vi "Get Child Channels.vi"(7 "Channel Type":T1, 8 "error in":errorcluster, 11 "Section Ref in":T2 format="%.0x") -> (0 "error out":errorcluster, 2 "Channel Refs":T2[](array[typedef]) format="%.0x", 3 "Section Ref out":T2 format="%.0x", 4 "Found":bool)   [LabVIEW 2020, in "SEECD Engine.lvlib"]
doc: "Returns an array of channel references for all the channels within the section specified by Section Ref in. This array includes references to both input and output channels.\n\nThis function performs a depth-first deep search for channels in the hierarchy."
uses:
  SEECD Engine.lvlib
  <vilib>/NI VeriStand/Custom Device API/Custom Device Item Ref.ctl
  <vilib>/NI VeriStand/Custom Device API/Custom Device Channel Type.ctl
  <vilib>/NI VeriStand/Custom Device API/Custom Device API.lvlib
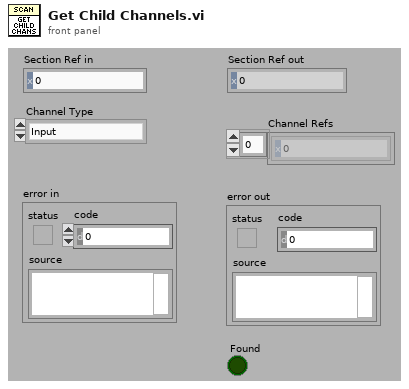
[diagram p1: front panel]
types:
  T1 = typedef "Custom Device API.lvlib/Custom Device Channel Type.ctl" = enum16{"Input", "Output"}
  T2 = typedef "Custom Device API.lvlib/Custom Device Item Ref.ctl" = u64
  T3 = typedef "Custom Device API.lvlib/Custom Device Item Info.ctl" = cluster{"Name":string, "Is Channel":bool, "GUID":string, "Is Waveform":bool}
  T4 = typedef "Custom Device API.lvlib/Custom Device Channel.ctl" = cluster{"Type":T1, "Units":string, "Default Value":dbl, "Faultable":bool, "Scalable":bool}
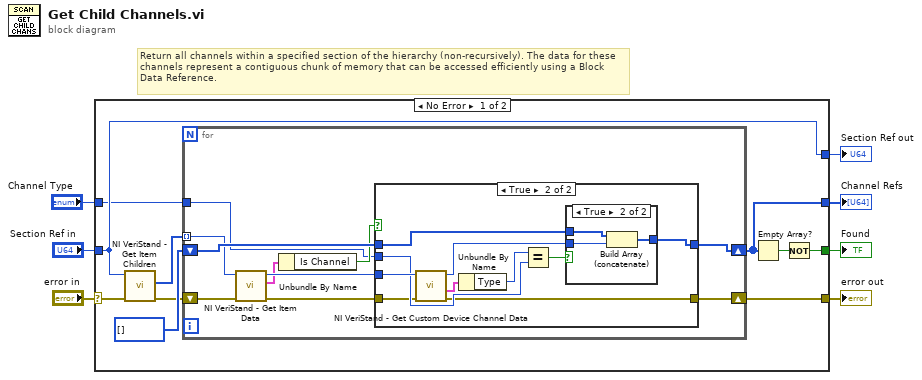
[diagram p0: block diagram]
diagram:
  # "Return all channels within a specified section of the hierarchy (non-recursively). The data for these channels represent a contiguous chunk of memory that can be accessed efficiently using a Block Data Reference."
  n1 = case shown="No Error" "error in" {
    selector: "error in" -> [w9 w45]
    tunnel: "Section Ref in" -> [w12 w44]
    tunnel: [w17 w45] -> w6
    tunnel: [w15 _] -> w5
    tunnel: [w13 _] -> w4
    tunnel: [w12 w44] -> w2
    tunnel: "Channel Type" -> [w10 _]
    frame No Error {
      n2 = call <vilib>:"NI VeriStand - Get Item Children.vi"("error in (no error)"=w9, "Item Ref in"=w12) -> ("error out"=w8:errorcluster, "Child Refs"=w11:T2[])  [unwired: 8 out]
      n3 = for {
        shift-right: [w18] -> w17
        shift-left: w8 -> [w27]
        shift-right: [w25] -> w15
        shift-left: T2[] [] ("appended array") -> [w26]
        tunnel: w11 -> [w21] mode=indexing
        tunnel: w10 -> [w20]
        n4 = call <vilib>:"NI VeriStand - Get Item Data.vi"("error in (no error)"=w27, "Item Ref in"=w21) -> ("error out"=w19:errorcluster, "Item Info"=w23:T3, "Item Ref out"=w24:T2)  [unwired: 7 out]
        n5 = Unbundle By Name(w23) -> ("Is Channel"=w22:bool)
        n6 = case shown="True" w22 {
          tunnel: w26 -> [w29 w39]
          tunnel: [w29 w38] -> w25
          tunnel: w24 -> [_ w37]
          tunnel: w20 -> [_ w34]
          tunnel: w19 -> [w28 w31]
          tunnel: [w28 w30] -> w18
          frame False {
          }
          frame True {
            n7 = call <vilib>:"NI VeriStand - Get Custom Device Channel Data.vi"("error in (no error)"=w31, "Channel Ref in"=w37) -> ("error out"=w30:errorcluster, "Channel"=w36:T4, "Channel Ref out"=w32:T2)  [unwired: 4 in, 3 out]
            n8 = Unbundle By Name(w36) -> ("Type"=w35:T1)
            n9 = Equal?(x=w35, y=w34) -> (x = y?=w33:bool)
            n10 = case shown="True" w33 {
              tunnel: w39 -> [w40 w43]
              tunnel: [w40 w42] -> w38
              tunnel: w32 -> [_ w41]
              frame False {
              }
              frame True {
                n11 = Build Array (concatenate)(w43, w41) -> (w42:T2[])
              }
            }
          }
        }
      }
      n12 = Empty Array?(array=w15) -> (empty?=w14:bool)
      n13 = Not(x=w14) -> (.not. x?=w13:bool)
    }
    frame Error {
    }
  }
  "Found" <- w4
  "error out" <- w6
  "Section Ref out" <- w2
  "Channel Refs" <- w5
